vi "Build user folder path.vi"() -> (3 "Daily folder path with user folder appended?":path)   [LabVIEW 2020]
uses:
  Global Variables/General Globals.vi
  User Interface/User profiles code/Globals/gl_UsrProfiles globals.vi
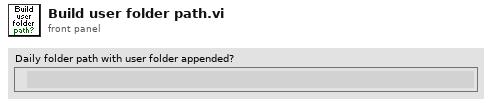
[diagram p1: front panel]
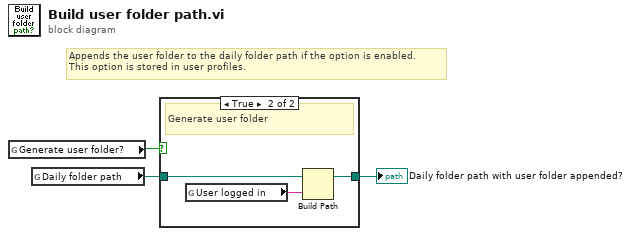
[diagram p0: block diagram]
diagram:
  # "Appends the user folder to the daily folder path if the option is enabled.\nThis option is stored in user profiles."
  n1 = global read "General Globals.vi" "Generate user folder?"() -> (w2:bool)
  n2 = global read "General Globals.vi" "Daily folder path"() -> (w1:path)
  n3 = case shown="True" w2 {
    tunnel: w1 -> [w4 w7]
    tunnel: [w4 w6] -> w3
    frame False {
      # "Do not generate user folder"
    }
    frame True {
      # "Generate user folder"
      n4 = global read "gl_UsrProfiles globals.vi" "User logged in"() -> (w5:string)
      n5 = Build Path(base path=w7, name or relative path=w5) -> (appended path=w6:path)
    }
  }
  "Daily folder path with user folder appended?" <- w3
